vi "Get STATUS.vi"(8 "error in (no error)":errorcluster, 11 "VISA Refnum in":refnum<visa-resource-name>) -> (0 "error out":errorcluster, 1 "Read value":string, 2 "LED ON":bool, 3 "VISA Refnum out":refnum<visa-resource-name>)   [LabVIEW 2023]
uses:
  5fd05b91-fe5d-4e4b-a27d-734f00cc7743.vi
  Serial_communication.lvlib
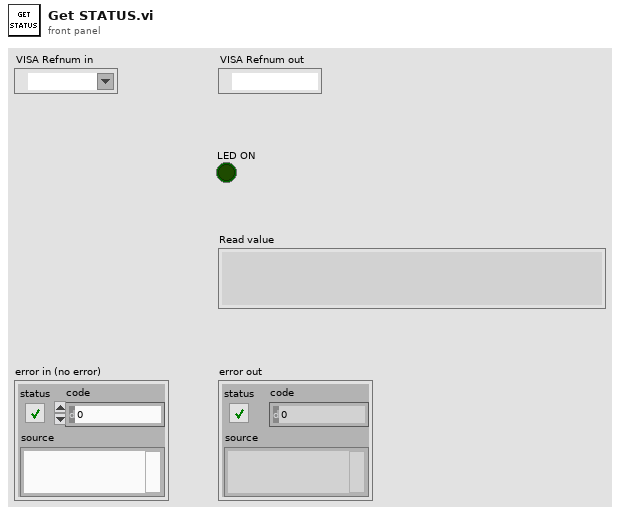
[diagram p1: front panel]
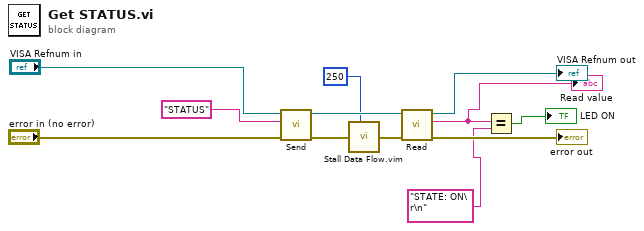
[diagram p0: block diagram]
diagram:
  n1 = call "Send.vi"("error in (no error)"="error in (no error)", "Command"="STATUS", "VISA Refnum in"="VISA Refnum in") -> ("error out"=w9:errorcluster, "VISA Refnum out"=w10:refnum<visa-resource-name>)  [unwired: 7 in]
  n2 = call "Stall Data Flow.vim"("value in"=w9, "milliseconds to wait"=u32 250) -> ("value out"=w8:errorcluster)  [unwired: 1 out]
  n3 = call "Read.vi"("error in (no error)"=w8, "VISA Refnum in"=w10) -> ("error out"=→"error out":errorcluster, "Read value"=w2:string, "VISA Refnum out"=→"VISA Refnum out":refnum<visa-resource-name>)  [unwired: 7 in]
  "Read value" <- w2
  n4 = Equal?(x=w2, y="STATE: ON\r\n" ("Read value 2")) -> (x = y?=→"LED ON":bool)
